vi "Listbox - Complete.vi"(7 "Row to Update":i32, 8 "error in (no error)":errorcluster, 11 "SV B-M In":refnum<class "SV B-M (Host).lvclass">) -> (0 "error out":errorcluster, 3 "SV B-M Out":refnum<class "SV B-M (Host).lvclass">)   [LabVIEW 2015, in "SV B-M (Host).lvclass"]
doc: "Updates a specific line in the listbox when a phase has been completed. Displays success or error and fills the elapsed time."
uses:
  SV B-M (Host).lvclass
  SV B-M (Host).lvclass/SV B-M (Host).ctl
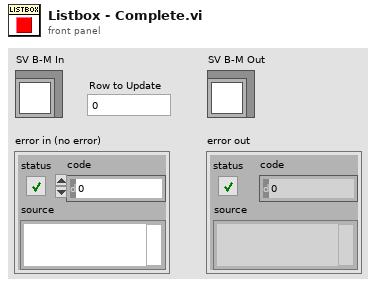
[diagram p1: front panel]
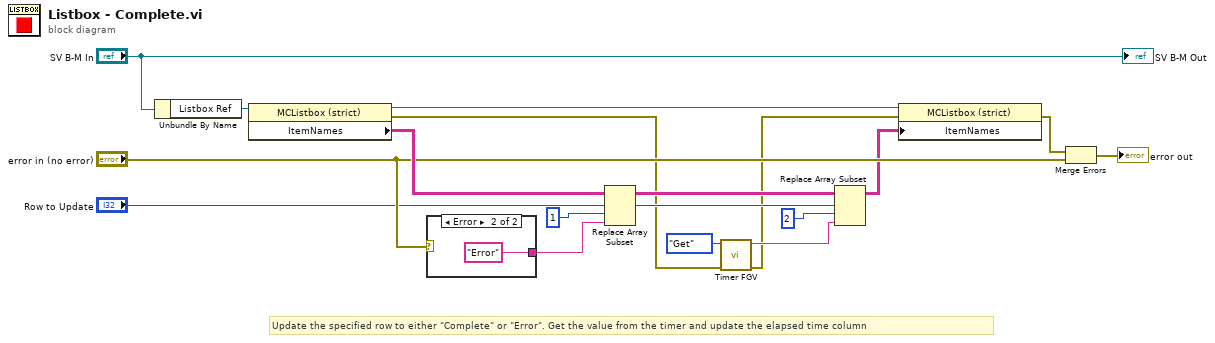
[diagram p0: block diagram]
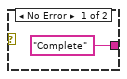
[diagram p2: hidden frame]
diagram:
  # "Update the specified row to either \"Complete\" or \"Error\". Get the value from the timer and update the elapsed time column"
  n1 = Unbundle By Name("SV B-M In") -> ("Listbox Ref"=w16:refnum<vi>)
  n2 = property on="Property Node" class="MCListbox (strict)"(reference=w16) -> (reference out=w17:refnum<vi>, error out=w3:errorcluster, "ItemNames"=w13:string[][])  [unwired: 1 in]
  n3 = case shown="Error" "error in (no error)" {
    tunnel: ["Complete" "Error"] -> w10
    frame No Error {
    }
    frame Error {
    }
  }
  n4 = Replace Array Subset(array=w13, new element=w10, index (row)="Row to Update", index (col)=1 ("disabled index (col)")) -> (w7:string[][])
  n5 = call "Timer FGV.vi"("error in (no error)"=w3, "Mode"=enum16{"Set", "Get"}."Get") -> ("error out"=w2:errorcluster, "Elapsed Time (sec)"=w4:string)  [unwired: 8 in]
  n6 = Replace Array Subset(array=w7, new element=w4, index (row)="Row to Update", index (col)=2 ("disabled index (col)")) -> (w1:string[][])
  n7 = property class="MCListbox (strict)"(reference=w17, error in=w2, "ItemNames"=w1) -> (error out=w9:errorcluster)  [unwired: 1 out]
  n8 = Merge Errors(w9, "error in (no error)") -> (→"error out":errorcluster)
  "SV B-M Out" <- "SV B-M In"
